vi "Start Stream.vi"(8 "error in (no error)":errorcluster, 11 "Pulse Driver in":refnum<class "Pulse Driver.lvclass">) -> (0 "error out":errorcluster, 3 "Pulse Driver out":refnum<class "Pulse Driver.lvclass">)   [LabVIEW 2016, in "Pulse Driver.lvclass"]
uses:
  Pulse Driver.lvclass
  C:/github/NHMFL_Core/Libraries/Instruments/Instrument Driver/Instrument Driver.lvclass
  Pulse Driver.lvclass/Pulse Driver.ctl
  Instrument Driver/Instrument Driver.lvclass/Instrument Driver.ctl
  Read Scaling coefficients.vi
  Read t0.vi
  Read dt.vi
  Read tdms file.vi
  Instrument Driver/Read Channel names.vi
  Instrument Driver/Read Group name.vi
  Write tdms file.vi
  <vilib>/Utility/tdmsutil.llb/TDMS Create Scaling Information (Linear).vi
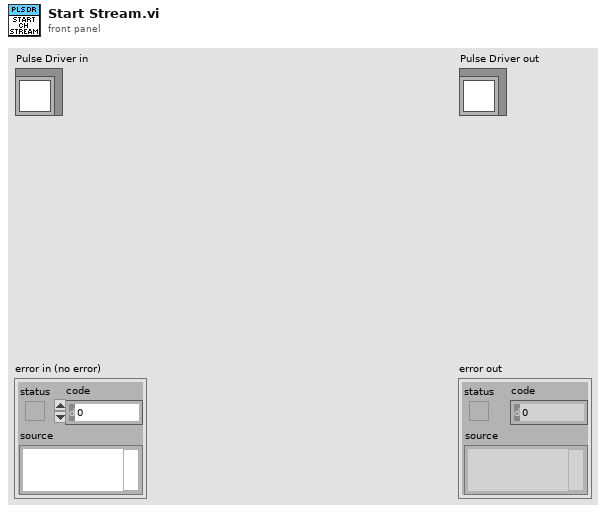
[diagram p1: front panel]
types:
  T1 = cluster{"slope":dbl, "y intercept":dbl, "input source":i32}
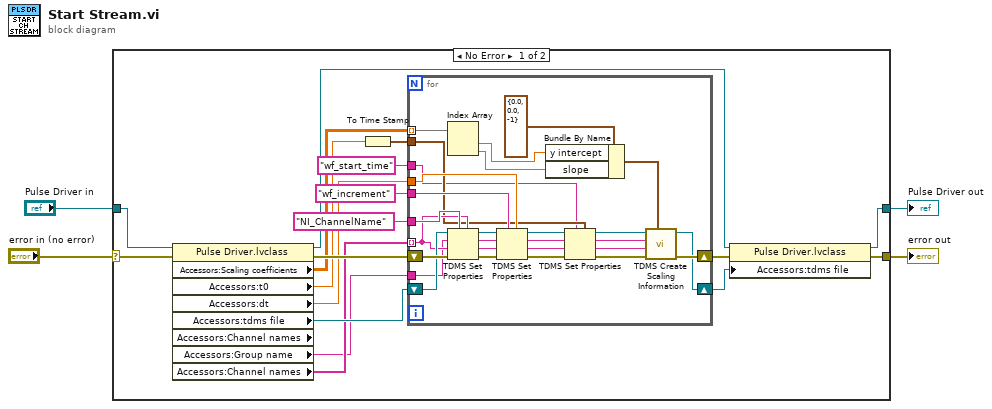
[diagram p0: block diagram]
diagram:
  n1 = case shown="No Error" "error in (no error)" {
    selector: "error in (no error)" -> [w14 w52]
    tunnel: [w15 w52] -> w3
    tunnel: [w18 w51] -> w1
    tunnel: "Pulse Driver in" -> [w22 w51]
    frame No Error {
      n2 = property class="Pulse Driver.lvclass" props=["Accessors:Scaling coefficients", "Accessors:t0", "Accessors:dt", "Accessors:tdms file", "Accessors:Channel names", "Accessors:Group name", "Accessors:Channel names"](reference=w22, error in=w14) -> (reference out=w21:refnum<class "Pulse Driver.lvclass">, error out=w20:errorcluster, "Accessors:Scaling coefficients"=w19:dbl[][], "Accessors:t0"=w8:dbl, "Accessors:dt"=w9:dbl, "Accessors:tdms file"=w13:refnum<k34>, "Accessors:Group name"=w5:string, "Accessors:Channel names"=w10:string[])  [unwired: 1 out]
      n3 = To Time Stamp(1:w8) -> (0:w7:timestamp)
      n4 = for {
        tunnel: w19 -> [w47] mode=indexing
        tunnel: "NI_ChannelName" -> [w40]
        tunnel: w10 -> [w39] mode=indexing
        tunnel: w9 -> [w38]
        tunnel: w7 -> [w37]
        tunnel: "wf_start_time" -> [w36]
        shift-right: [w45] -> w17
        shift-left: w20 -> [w48]
        shift-right: [w44] -> w16
        shift-left: w13 -> [w42]
        tunnel: "wf_increment" -> [w41]
        tunnel: w5 -> [w25]
        n5 = Index Array(array=w47) -> (element #1=w50:dbl, element #2=w43:dbl)  [unwired: 2 in]
        n6 = TDMS Set Properties(5:w39, 7:w40, 8:w48, 9:w39, 10:w25, 11:w42) -> (0:w35:errorcluster, 1:w32:string, 2:w34:string, 3:w33:refnum<k34>)
        n7 = TDMS Set Properties(5:w38, 7:w41, 8:w35, 9:w32, 10:w34, 11:w33) -> (0:w31:errorcluster, 1:w30:string, 2:w29:string, 3:w28:refnum<k34>)
        n8 = Bundle By Name(cluster=T1 {"slope"=0.0, "y intercept"=0.0, "input source"=-1} ("linear scale"), "y intercept"=w50, "slope"=w43) -> (w49:T1)
        n9 = TDMS Set Properties(5:w37, 7:w36, 8:w31, 9:w30, 10:w29, 11:w28) -> (0:w27:errorcluster, 1:w23:string, 2:w24:string, 3:w26:refnum<k34>)
        n10 = call-poly <vilib>:"TDMS Create Scaling Information.vi"("linear scale"=w49, "error in (no error)"=w27, "channel name"=w23, "group name"=w24, "tdms file"=w26) -> ("error out"=w45:errorcluster, "tdms file out"=w44:refnum<k34>)  [unwired: 2 in, 3 out]
      }
      n11 = property class="Pulse Driver.lvclass"(reference=w21, error in=w17, "Accessors:tdms file"=w16) -> (reference out=w18:refnum<class "Pulse Driver.lvclass">, error out=w15:errorcluster)
    }
    frame Error {
    }
  }
  "error out" <- w3
  "Pulse Driver out" <- w1
